vi "5-InitialAllHardware.vi"(8 "error in (no error)":errorcluster, 11 "AllControls IN":T1) -> (3 "InitalResult":bool[](array[boolean]))   [LabVIEW 2017]
uses:
  Ctrls/AllControls.ctl
panel:
  out "error out":errorcluster
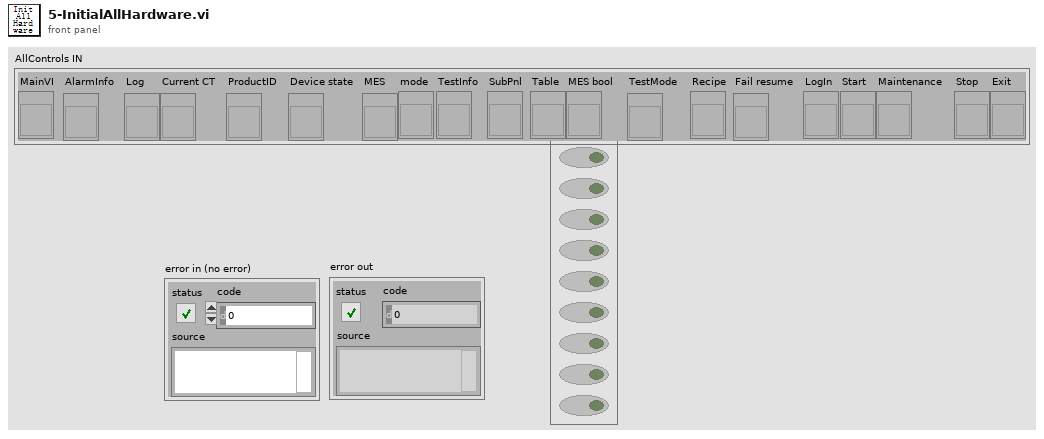
[diagram p1: front panel]
types:
  T1 = typedef "AllControls.ctl" = cluster{"MainVI":refnum<vi>, "AlarmInfo":refnum<vi>, "Log":refnum<vi>, "Current CT":refnum<vi>, "ProductID":refnum<vi>, "Device state":refnum<vi>, "MES":refnum<vi>, "mode":refnum<vi>, "TestInfo":refnum<vi>, "SubPnl":refnum<vi>, "Table":refnum<vi>, "MES bool":refnum<vi>, "TestMode":refnum<vi>, "Recipe":refnum<vi>, "Fail resume":refnum<vi>, "LogIn":refnum<vi>, "Start":refnum<vi>, "Maintenance":refnum<vi>, "Stop":refnum<vi>, "Exit":refnum<vi>}
  T2 = typedef "HD Config.ctl" = cluster{" PC":cluster{"PC Address":u8[], "PC Port":i32}, "FCO":cluster{"COM":refnum<visa-resource-name>, "Baudrate":u32}, "DC Power ":cluster{"COM":refnum<visa-resource-name>, "Baudrate":u32}, "PW3336":cluster{"COM":refnum<visa-resource-name>, "Baudrate":u32}, "Lefoo":cluster{"COM":refnum<visa-resource-name>, "Baudrate":u32}, "AI Model":cluster{"COM":refnum<visa-resource-name>, "Baudrate":u32}, "DIPC":cluster{"COM":refnum<visa-resource-name>}, "RFID":cluster{"IP Address":string, "Port":u16, "Retry":u16}, "Motor":cluster{"COM":refnum<visa-resource-name>, "Baudrate":u32}, "Fail_resume_mode":bool, "GRR":bool}
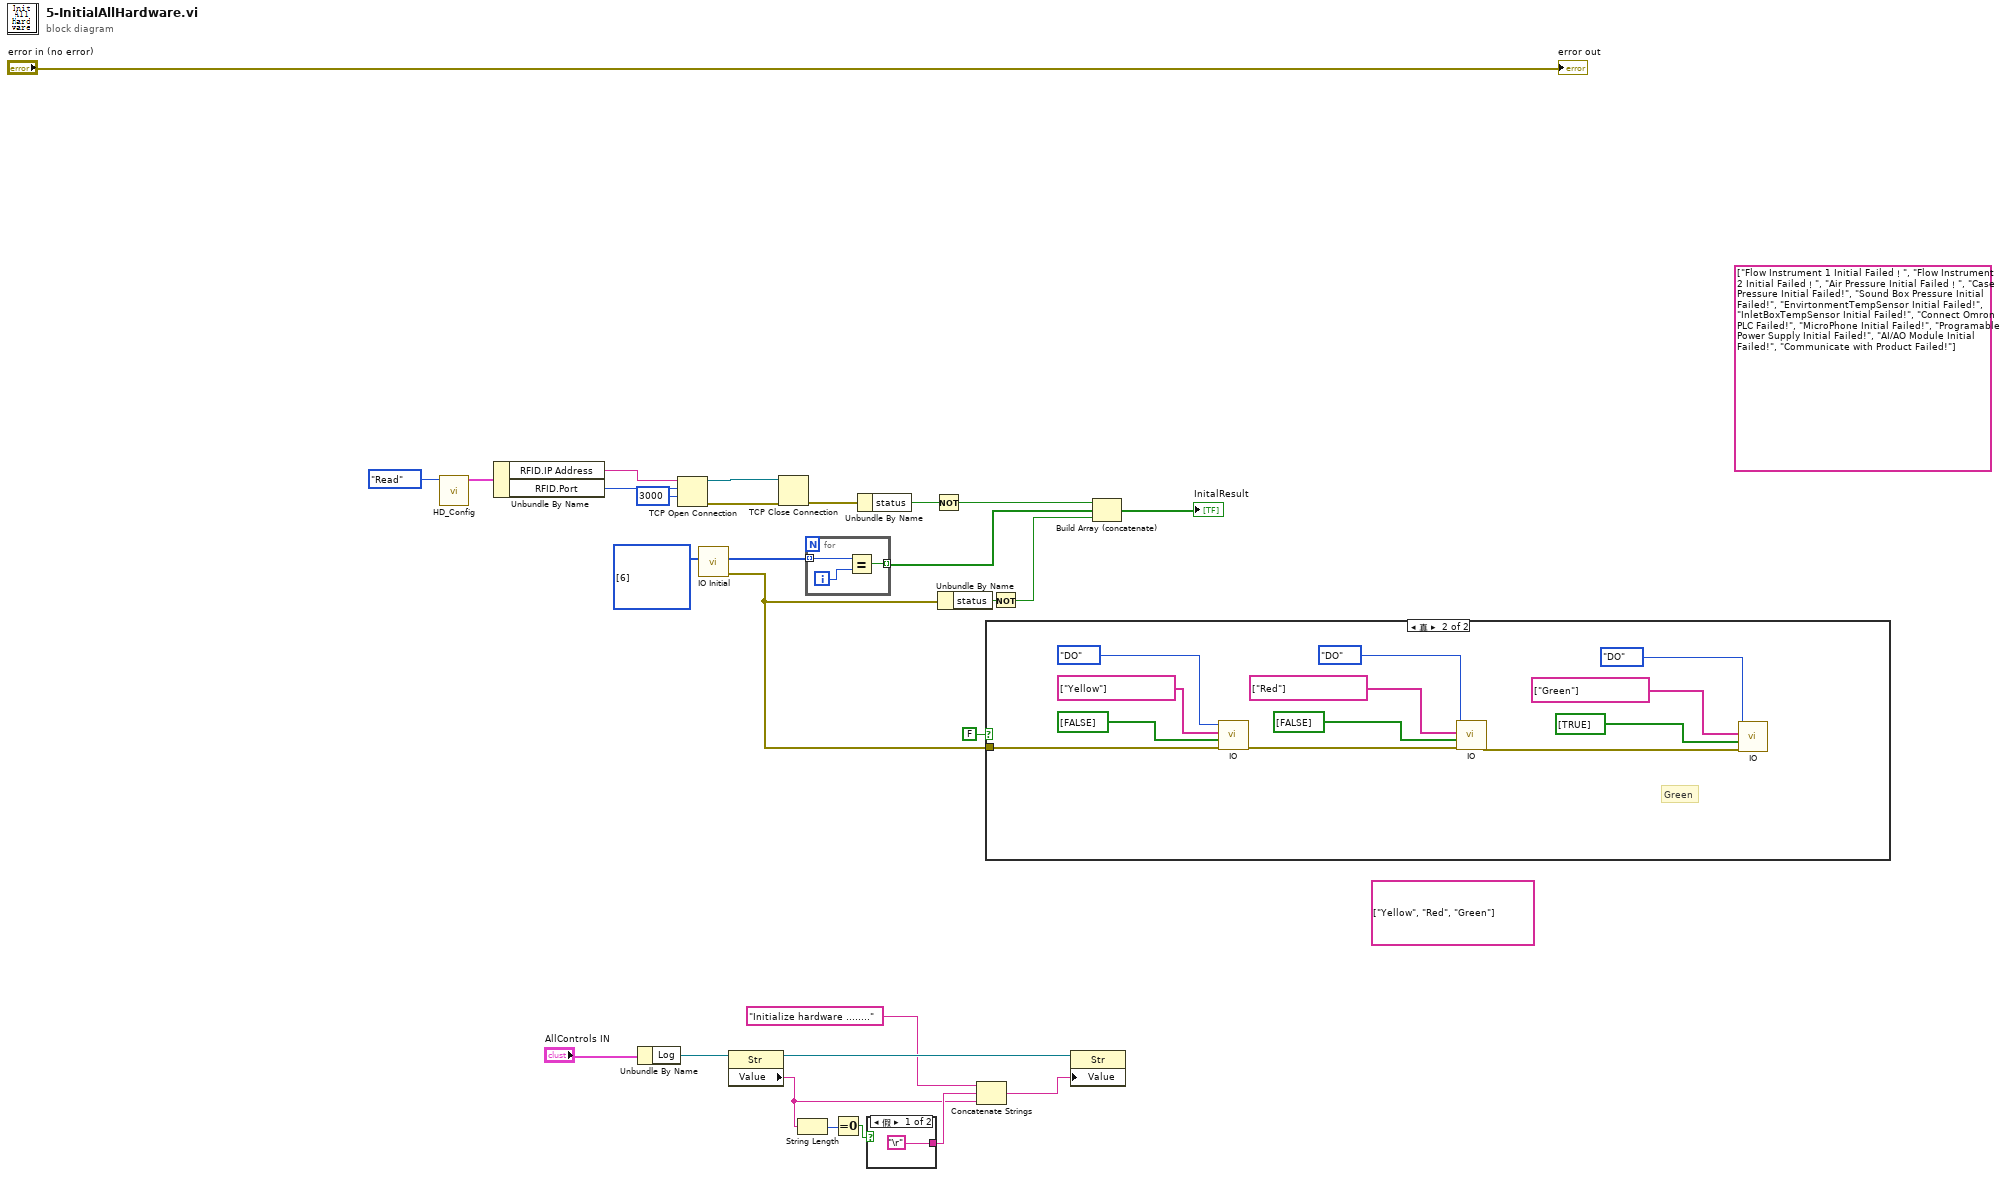
[diagram p0: block diagram]
diagram:
  (unwired) string[] ["Yellow", "Red", "Green"] ("IO Name")
  w21 = u16[] [6] items=["PCI-7230"=6, "PCI-7432"=16, "PCI-7433"=17, "PCI-7434"=18, "PCI-7442"=37] ("CardType")
  (unwired) string[] ["Flow Instrument 1 Initial Failed！", "Flow Instrument 2 Initial Failed！", "Air Pressure Initial Failed！", "Case Pressure Initial Failed!", "Sound Box Pressure Initial Failed!", "EnvirtonmentTempSensor Initial Failed!", "InletBoxTempSensor Initial Failed!", "Connect Omron PLC Failed!", "MicroPhone Initial Failed!", "Programable Power Supply Initial Failed!", "AI/AO Module Initial Failed!", "Communicate with Product Failed!"]
  n1 = call "HD_Config.vi"("Step"=enum16{"Initial", "Write", "Read"}."Read") -> ("HD Config out"=w25:T2)  [unwired: 9 in, 1 out]
  n2 = Unbundle By Name(w25) -> ("RFID.IP Address"=w9:string, "RFID.Port"=w24:u16)
  n3 = Unbundle By Name("AllControls IN") -> ("Log"=w16:refnum<vi>)
  n4 = TCP Open Connection(address=w9, remote port or service name=w24, timeout ms (60000)=3000 ("超时毫秒(60000)")) -> (connection ID=w5:refnum<k5>, error out=w4:errorcluster)  [unwired: 2 in]
  n5 = call "IO Initial.vi"("CardType"=w21) -> ("error out"=w2:errorcluster, "IO f"=w20:i16[])  [unwired: 9 in]
  n6 = property class="Str"(reference=w16) -> (reference out=w18:refnum<vi>, "Value"=w11:string)  [unwired: 1 in, 1 out]
  n7 = TCP Close Connection(connection ID=w5, error in (no error)=w4) -> (error out=w3:errorcluster)  [unwired: 1 in, 1 out]
  n8 = String Length(string=w11) -> (length=w13:i32)
  n9 = for {
    tunnel: w20 -> [w31] mode=indexing
    tunnel: [w29] -> w7 mode=indexing
    i -> [w30]
    n10 = Equal?(x=w31, y=w30) -> (x = y?=w29:bool)
  }
  n11 = Equal To 0?(x=w13) -> (x = 0?=w14:bool)
  n12 = Unbundle By Name(w3) -> ("status"=w22:bool)
  n13 = case shown="假" w14 {
    tunnel: ["\r" _] -> w12
    frame False {
    }
    frame True {
    }
  }
  n14 = Not(x=w22) -> (.not. x?=w8:bool)
  n15 = Unbundle By Name(w2) -> ("status"=w19:bool)
  n16 = Concatenate Strings("Initialize hardware ........" ("字符串"), w12, w11) -> (w15:string)
  n17 = case shown="真" FALSE {
    tunnel: w2 -> [_ w44]
    frame False {
    }
    frame True {
      # "Green"
      n18 = call "IO.vi"("错误常量"=w44, "DO DATA"=bool[] [FALSE], "IO Name"=string[] ["Yellow"], "IO?"=enum16{"DI", "DO"}."DO") -> ("error out"=w34:errorcluster)  [unwired: 5 in, 2 out]
      n19 = call "IO.vi"("错误常量"=w34, "DO DATA"=bool[] [FALSE], "IO Name"=string[] ["Red"], "IO?"=enum16{"DI", "DO"}."DO") -> ("error out"=w33:errorcluster)  [unwired: 5 in, 2 out]
      n20 = call "IO.vi"("错误常量"=w33, "DO DATA"=bool[] [TRUE], "IO Name"=string[] ["Green"], "IO?"=enum16{"DI", "DO"}."DO") -> ()  [unwired: 5 in, 3 out]
    }
  }
  n21 = Not(x=w19) -> (.not. x?=w6:bool)
  n22 = property class="Str"(reference=w18, "Value"=w15) -> ()  [unwired: 1 in, 2 out]
  n23 = Build Array (concatenate)(w8, w7, w6) -> (→"InitalResult":bool[])
  "error out" <- "error in (no error)"
